vi "decimate.vi"(10 "Sample Group Size":i64, 11 "Array in":dbl[](array[numeric])) -> (3 "Array out":dbl[](array[numeric]))   [LabVIEW 2025, in "LabJackEKG.lvlib"]
uses:
  LabJackEKG.lvlib
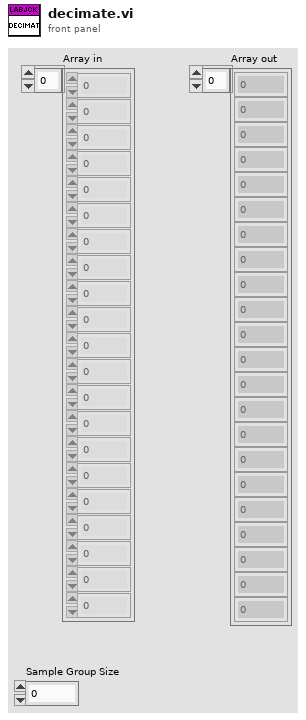
[diagram p1: front panel]
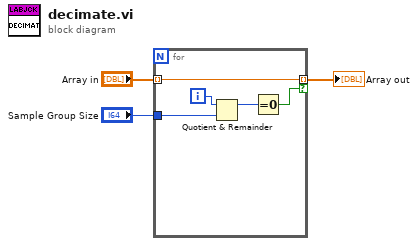
[diagram p0: block diagram]
diagram:
  n1 = for {
    tunnel: "Array in" -> [w8] mode=indexing
    tunnel: [w8] -> w2 mode=indexing if=w4
    tunnel: "Sample Group Size" -> [w6]
    i -> [w7]
    n2 = Quotient & Remainder(x=w7, y=w6) -> (x-y*floor(x/y)=w5:i64)  [unwired: 1 out]
    n3 = Equal To 0?(x=w5) -> (x = 0?=w4:bool)
  }
  "Array out" <- w2
